vi "X-Pixel.vi"() -> ()   [LabVIEW 2018]
panel:
  out "X-Pixel":dbl
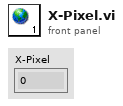
[diagram p1: front panel]
diagram:
